vi "RandomLaser.vi"() -> ()   [LabVIEW 2014]
doc: "Random Laser Project\nAndré Romero - 2020\nandretec@ifsc.usp.br\n\nMain Program"
uses:
  OceanOptics.ctl
  PowerMeterSteps.ctl
  RL-Signal.ctl
  <vilib>/Analysis/2dsp.llb/Integral Method.ctl
  <vilib>/Analysis/8numeric.llb/1D Numeric Integration.vi
  GlobalVariables.vi
  <vilib>/Utility/file.llb/Write To Spreadsheet File (DBL).vi
  <vilib>/Analysis/NI_AAL_SigProc.lvlib
  <vilib>/Analysis/NI_AALBase.lvlib
  <vilib>/Analysis/NI_AALPro.lvlib
panel:
  out "delta WL":dbl=0.38690207279938704
  in  "Stop":bool
  out "Power Meter":dbl[](array[numeric])=[-0.0003675591076923077, -0.0002657142871794872, -0.00022899957179487178, 0.00042243897435897433, 0.0004997026012820513, 0.0006796630115384615, 0.000805894673076923, 0.0010408828243589744, 0.0018024533846153848, 0.0023367831153846153, 0.0029247413076923076, 0.0028397148461538463, 0.003205695884615385, 0.0036658875128205127, 0.003961987641025641, 0.004680868307692308, 0.005090419641025641, 0.006488342294871795, 0.007851225423076924, 0.007202216717948717, 0.008655850807692307, 0.008092802884615384, 0.009669394692307692, 0.008936860974358975, 0.009809811717948718, 0.010228137487179488, 0.011672985217948718, 0.012192949025641026, 0.011663994371794871, 0.012874870384615385, 0.01270935917948718, 0.014818592820512821, 0.016178746282051282, 0.016049180384615384, 0.0160890691025641, 0.014186609871794872]
  out "Spectrum":dbl[][](array[numeric])
  out "Amplitudes":dbl[](array[numeric])=[0.0, 0.0, 0.0, 0.0, 0.0, 0.0, 0.0, 0.0, 0.0, 5575.9914689081015, 6701.8830329298, 8561.647140939602, 9059.66238048701, 10013.63040535748, 10875.931356857935, 12579.417450238643, 13233.340345584173, 16127.947959725754, 16741.788066185352, 19933.198034888228, 18892.002085463362, 24420.615194539, 23300.805099557427, 26519.160159321964, 32440.49170739598, 32440.49170739598, 34903.27520346824, 42840.78445676197, 42414.61716171854, 40488.768647175595, 43435.97106846481, 43435.97106846481, 51858.85499836823, 55040.55736237094, 56733.873142532764, 55752.38318456956]
  out "Locations Peaks":dbl[](array[numeric])=[0.0, 0.0, 0.0, 0.0, 0.0, 0.0, 0.0, 0.0, 0.0, 624.9085485139512, 623.199026880973, 622.8569840323327, 622.514895045022, 623.199026880973, 623.199026880973, 622.514895045022, 622.8569840323327, 622.514895045022, 622.8569840323327, 622.514895045022, 622.8569840323327, 622.514895045022, 622.8569840323327, 622.8569840323327, 622.8569840323327, 622.8569840323327, 622.514895045022, 622.514895045022, 622.8569840323327, 622.8569840323327, 622.8569840323327, 622.8569840323327, 622.8569840323327, 622.8569840323327, 622.8569840323327, 622.8569840323327]
  out "Integration":dbl[](array[numeric])=[93876.86248643893, 89574.62293993768, 89574.62293993768, 92418.20959135504, 106316.38021475376, 190489.0806594419, 173427.09120228325, 190883.0319805349, 253633.0446140827, 281236.16658956936, 317841.71014271444, 374352.8298044355, 395197.03367327957, 421997.2274496375, 457040.3478550627, 509121.0411876146, 518774.7267490108, 600545.4510518024, 620849.4391936888, 726021.5293375205, 667303.2962255043, 857398.8951125076, 805420.7981609555, 876101.0180196995, 973816.9103050136, 973816.9103050136, 1101330.125428112, 1300810.123723178, 1183680.9770934903, 1213324.5227469385, 1256065.8933422558, 1256065.8933422558, 1483869.301248752, 1539653.32481904, 1616784.6736414272, 1629926.8709311432]
  out "size(s)":i32=109
  out "Waveform Graph 2":dbl[](graph)=[-0.005487304474358975, -0.005832730371794871, -0.0058483878589743596, -0.0058483878589743596, -0.005573613, -0.005095886692307692, -0.004915247423076923, -0.004803107, -0.004803107, -0.00415237408974359, -0.003636093397435897, -0.003279903192307692, -0.003279903192307692, -0.002614101384615385, -0.002614101384615385, -0.0017563094487179488, -0.0017563094487179488, -0.0006636677525641026, -0.00025933357564102567, -0.00025933357564102567, 0.0005514882038461538, 0.0005514882038461538, 0.001194198632051282, 0.0014312010128205129, 0.0014312010128205129, 0.0027755268974358977, 0.003001960487179487, 0.003001960487179487, 0.003652692653846154, 0.004357635564102564, 0.0060297748717948714, 0.0060297748717948714, 0.006476770166666666, 0.0073061897820512825, 0.008219170974358975, 0.008605500435897437, 0.008900238666666666, 0.010023608461538462, 0.010305812628205128, 0.010305812628205128, 0.012418297, 0.012980169615384615, 0.014193191923076921, 0.013533851282051281, 0.013533851282051281, 0.014171850512820513, 0.01582010935897436, 0.018513849487179487, 0.018513849487179487, 0.020606362692307693, 0.02333670346153846, 0.02333670346153846, 0.022893022307692308, 0.02429118076923077, 0.02429118076923077, 0.02647001435897436, 0.02670231076923077, 0.02670231076923077, 0.027472030897435898, 0.02830790782051282, 0.02830790782051282, 0.02888465923076923, 0.03174886423076923, 0.03174886423076923, 0.032283935897435896, 0.03257239217948718, 0.03271840076923077, 0.03444572064102564, 0.034723633846153845, 0.034723633846153845, 0.03663491371794872, 0.03663491371794872, 0.03613761141025641, 0.03828260551282051, 0.03805538666666667, 0.03805538666666667, 0.03951163782051282, 0.04004338717948718, 0.039338835769230765, 0.039338835769230765, 0.04283988615384615, 0.042323017051282046, 0.042323017051282046, 0.04017059935897436, 0.04026514051282051, 0.041000410641025636, 0.041000410641025636, 0.04617789256410257, 0.04617789256410257, 0.046548361923076924, 0.04826218653846154, 0.04826218653846154, 0.048524028461538464, 0.04702962294871795, 0.04661353666666666, 0.04663584961538462, 0.04663584961538462, 0.0458491058974359, 0.04640453230769231, 0.04640453230769231, 0.04648593948717949, 0.04691024641025641, 0.04691024641025641, 0.04794475782051282, 0.04896243064102564, 0.05036391884615385, 0.05036391884615385, 0.04973549115384615, 0.04851584358974359]
  out "Motor Target":i32
  out "step error":dbl=4.6948184809657505
  out "Numeric Control":i32=571
  out "appended array":dbl[](array[numeric])=[0.03814716076923077, 0.04028040576923077, 0.03893296115384615, 0.03881278179487179, 0.03962595474358974, 0.03962595474358974, 0.04072623166666667, 0.042531442307692305, 0.042531442307692305, 0.04118947217948718, 0.04118947217948718, 0.043604905, 0.04170907846153846, 0.047686999358974365, 0.04542324666666667, 0.04744549717948718, 0.04744549717948718, 0.04903151871794872, 0.04903151871794872, 0.05148572076923077, 0.05148572076923077, 0.04996409794871795, 0.04996409794871795, 0.05131271576923077, 0.052321403717948724, 0.05075768333333334, 0.0506429873076923, 0.05160921064102564, 0.04980653423076923, 0.04980653423076923, 0.05041557743589743, 0.050435350128205124, 0.05207693756410257, 0.0510150267948718, 0.04899962987179487, 0.05028836243589744, 0.05107413, 0.05107413, 0.047357233589743586, 0.05035041474358974, 0.050845735, 0.050845735, 0.049560324871794875, 0.049386343589743587, 0.049386343589743587, 0.0474762308974359, 0.05124815, 0.05124815, 0.04991651987179487, 0.047606959358974354, 0.046334271153846154, 0.047763528974358975, 0.047946701025641025, 0.04803633192307692, 0.04881388474358974, 0.04784396294871795, 0.04784396294871795, 0.04528820487179487, 0.04316417756410257, 0.04157324871794872, 0.04189031333333333, 0.04189031333333333, 0.042249424743589746, 0.042249424743589746, 0.04073130923076923, 0.038956053205128204, 0.038956053205128204, 0.04025163923076923, 0.040992975, 0.03823464833333333, 0.037050615, 0.03659950551282051, 0.035411361794871796, 0.035411361794871796, 0.0335793308974359, 0.032886507564102566, 0.032659309615384616, 0.031678015000000004, 0.031678015000000004, 0.030108811153846154, 0.030108811153846154, 0.02815076512820513, 0.027613132307692308, 0.02745461641025641, 0.02745461641025641, 0.024971846153846153, 0.023404218333333334, 0.023404218333333334, 0.022565616153846155, 0.021971435384615386, 0.021303487435897436, 0.020184618333333335, 0.019698665, 0.019698665, 0.01710024217948718, 0.016112891025641025, 0.016112891025641025, 0.01559681141025641, 0.01566960833333333, 0.014254835256410258, 0.01331249358974359, 0.01331249358974359, 0.01175093273076923, 0.011184945320512821, 0.010219515294871796, 0.009239205, 0.008537592243589744, 0.008537592243589744, 0.008233652730769231, 0.007168407769230769, 0.007049413397435898, 0.006302984474358974, 0.0051921379102564105, 0.00454199676923077, 0.003954869897435898, 0.003954869897435898, 0.0031781009743589743, 0.0031781009743589743, 0.0029140872564102564, 0.0014977446794871795, 0.0014977446794871795, 0.0006180309871794871, -0.0002421096346153846, -0.0002421096346153846, -0.0010443222076923077, -0.0010443222076923077, -0.0019091590384615385, -0.0027440524102564103, -0.0027949365512820513, -0.0028524740769230767, -0.003429424858974359, -0.0048430307435897435, -0.004761224730769231, -0.004563362333333334, -0.004991378192307692, -0.004588804679487179, -0.004029664871794872, -0.003666037141025641, -0.003666037141025641, -0.003410441705128205, -0.002968921858974359, -0.002852083217948718, -0.002779084102564103, -0.002779084102564103, -0.002142247705128205, -0.0018751047564102563, -0.0018751047564102563, -0.0015238072564102564, -0.0011774021769230768, -0.0008895146423076923, -0.0006176758641025641, -0.00047911462564102563, -0.00047911462564102563, -0.0003826308576923077, -0.0013799610128205127, -0.0005440882743589744, -0.00013818675897435897, -0.00013818675897435897, 0.0018592164999999999, 0.0027060513974358972, 0.0034595305384615385, 0.0034595305384615385, 0.004154488961538461, 0.005114832538461538, 0.005114832538461538, 0.0064566116538461536, 0.006633336833333333, 0.006633336833333333, 0.006688135615384616, 0.007803289166666667, 0.007803289166666667, 0.009279321282051282, 0.009510256435897436, 0.009510256435897436, 0.010018718269230769, 0.011323302692307692, 0.013602139358974358, 0.013602139358974358, 0.014472458846153847, 0.014472458846153847, 0.015263318846153848, 0.016187063974358974, 0.01790519141025641, 0.01790519141025641, 0.019298054487179486, 0.019298054487179486, 0.020291468205128206, 0.020291468205128206, 0.021376090384615385, 0.021376090384615385, 0.02242841923076923, 0.023227692435897434, 0.025591651794871793, 0.025591651794871793, 0.026223805, 0.02971779294871795, 0.028628870897435897, 0.028628870897435897, 0.028008663717948717, 0.027696697564102566, 0.02956965, 0.02956965, 0.028673496794871793, 0.029780030384615387, 0.03213930923076923, 0.035217996025641025, 0.03527473807692308, 0.03527473807692308, 0.03669559897435897, 0.03665665358974359, 0.03785556128205128, 0.03754203987179487, 0.036888361794871795, 0.037945386153846156, 0.03861492346153846, 0.038500227435897434, 0.03922416064102564, 0.040526400384615385, 0.040526400384615385, 0.03986666282051282, 0.03986666282051282, 0.04169341923076923, 0.041507686025641026, 0.042650239743589745, 0.04226409, 0.04226409, 0.04266863628205128, 0.0441421408974359, 0.04573343076923077, 0.04521813487179487, 0.047250176153846156, 0.047250176153846156, 0.04542147653846154, 0.04631489551282051, 0.048990803205128206, 0.047789943333333335, 0.047789943333333335, 0.04684231358974359, 0.04454275576923077, 0.04685368358974359, 0.04762596192307692, 0.04675973038461539, 0.04675973038461539, 0.04527703205128205, 0.04527703205128205, 0.04157364871794872, 0.041092978846153844, 0.041092978846153844, 0.041301809999999994, 0.042665305, 0.04386481269230769, 0.04386481269230769, 0.04428675551282051, 0.0458058591025641, 0.046089819871794876, 0.046089819871794876, 0.046192972820512816, 0.0462835708974359, 0.044576599871794874, 0.044576599871794874, 0.04427247525641026, 0.04392391884615385, 0.04286120217948718, 0.04286120217948718, 0.04098240512820513, 0.04072601384615385, 0.03965080487179487, 0.03965080487179487, 0.0398696, 0.039303415641025644, 0.04005141987179487, 0.04017236935897436, 0.0395265241025641, 0.03754184576923077, 0.03754184576923077, 0.03593919487179487, 0.03592997423076923, 0.03364331756410256, 0.03334448538461539, 0.033942364615384614, 0.031980772435897434, 0.03136175038461538, 0.02979686871794872, 0.02979686871794872, 0.027415076923076924, 0.02804057653846154, 0.026967289871794874, 0.026967289871794874, 0.023854156153846156, 0.023854156153846156, 0.02363947141025641, 0.023173087692307692, 0.02205128576923077, 0.02286054987179487, 0.022448578461538464, 0.022448578461538464, 0.02149762794871795, 0.02094963717948718, 0.019584764487179485, 0.018592137307692307, 0.017544697948717946, 0.01551637141025641, 0.014312563846153847, 0.014088873333333331, 0.013259848461538461, 0.012367222012820513, 0.012367222012820513, 0.011250896833333333, 0.01044046858974359, 0.009141736282051283, 0.009141736282051283, 0.007557283448717949, 0.007557283448717949, 0.007006557628205129, 0.006270297884615385, 0.006270297884615385, 0.004901510038461538, 0.004901510038461538, 0.004756689756410257, 0.004255871782051282, 0.0034951461666666663, 0.0031088181794871796, 0.0025083835897435898, 0.0021981839615384615, 0.001356832141025641, 0.001356832141025641, 0.0003710442217948718, -0.00028144756666666665, -0.0007325553064102564, -0.0011335642525641025, -0.0011335642525641025, -0.001437696576923077, -0.0018406603717948718, -0.0018406603717948718, -0.002247147051282051, -0.002247147051282051, -0.0023632034230769232, -0.002725851705128205, -0.002725851705128205, -0.00294974317948718, -0.003120204871794872, -0.003120204871794872, -0.0034253148846153845, -0.0036460745256410255, -0.0055601084487179485, -0.005810028641025641, -0.00561432067948718, -0.005487304474358975, -0.005487304474358975, -0.005832730371794871, -0.0058483878589743596, -0.0058483878589743596, -0.005573613, -0.005095886692307692, -0.004915247423076923, -0.004803107, -0.004803107, -0.00415237408974359, -0.003636093397435897, -0.003279903192307692, -0.003279903192307692, -0.002614101384615385, -0.002614101384615385, -0.0017563094487179488, -0.0017563094487179488, -0.0006636677525641026, -0.00025933357564102567, -0.00025933357564102567, 0.0005514882038461538, 0.0005514882038461538, 0.001194198632051282, 0.0014312010128205129, 0.0014312010128205129, 0.0027755268974358977, 0.003001960487179487, 0.003001960487179487, 0.003652692653846154, 0.004357635564102564, 0.0060297748717948714, 0.0060297748717948714, 0.006476770166666666, 0.0073061897820512825, 0.008219170974358975, 0.008605500435897437, 0.008900238666666666, 0.010023608461538462, 0.010305812628205128, 0.010305812628205128, 0.012418297, 0.012980169615384615, 0.014193191923076921, 0.013533851282051281, 0.013533851282051281, 0.014171850512820513, 0.01582010935897436, 0.018513849487179487, 0.018513849487179487, 0.020606362692307693, 0.02333670346153846, 0.02333670346153846, 0.022893022307692308, 0.02429118076923077, 0.02429118076923077, 0.02647001435897436, 0.02670231076923077, 0.02670231076923077, 0.027472030897435898, 0.02830790782051282, 0.02830790782051282, 0.02888465923076923, 0.03174886423076923, 0.03174886423076923, 0.032283935897435896, 0.03257239217948718, 0.03271840076923077, 0.03444572064102564, 0.034723633846153845, 0.034723633846153845, 0.03663491371794872, 0.03663491371794872, 0.03613761141025641, 0.03828260551282051, 0.03805538666666667, 0.03805538666666667, 0.03951163782051282, 0.04004338717948718, 0.039338835769230765, 0.039338835769230765, 0.04283988615384615, 0.042323017051282046, 0.042323017051282046, 0.04017059935897436, 0.04026514051282051, 0.041000410641025636, 0.041000410641025636, 0.04617789256410257, 0.04617789256410257, 0.046548361923076924, 0.04826218653846154, 0.04826218653846154, 0.048524028461538464, 0.04702962294871795, 0.04661353666666666, 0.04663584961538462, 0.04663584961538462, 0.0458491058974359, 0.04640453230769231, 0.04640453230769231, 0.04648593948717949, 0.04691024641025641, 0.04691024641025641, 0.04794475782051282, 0.04896243064102564, 0.05036391884615385, 0.05036391884615385, 0.04973549115384615, 0.04851584358974359, 0.04851584358974359, 0.04918926448717949, 0.04918926448717949, 0.04768798435897436, 0.04749853782051282, 0.045149443846153846, 0.04514924974358975, 0.04693097435897436, 0.04693097435897436, 0.04631743282051282, 0.044912025256410255, 0.04394035730769231, 0.04564164179487179, 0.04489031230769231, 0.04489031230769231, 0.04320840641025641, 0.041405327051282054, 0.03952789717948718, 0.03952789717948718, 0.04017042025641026, 0.03891552269230769, 0.03727723974358974, 0.03727723974358974, 0.03708113961538462, 0.035381607307692305, 0.03470992666666667, 0.03470992666666667, 0.033015304615384614, 0.0317245991025641, 0.03036636948717949, 0.03337051474358974, 0.031271919615384614, 0.031271919615384614, 0.03185395435897436, 0.029991192820512817, 0.029809205769230768, 0.030315111025641026, 0.030740970128205126, 0.02854235935897436, 0.02854235935897436, 0.028143314487179487, 0.02606488012820513, 0.025311992435897435, 0.025311992435897435, 0.025301225512820512, 0.026598984615384614, 0.023089526923076923, 0.02366060076923077, 0.021547534358974357, 0.020616556538461537, 0.01807409358974359, 0.01857530782051282, 0.01828310987179487, 0.01758873730769231, 0.01758873730769231, 0.016613126153846153, 0.01586845166666667, 0.014894025512820513, 0.014096111923076924, 0.013694126794871794, 0.013694126794871794, 0.012646690423076925, 0.01233981964102564, 0.011144820089743589, 0.011144820089743589, 0.007031992141025642, 0.007031992141025642, 0.006841767269230769, 0.006366588282051282, 0.005964797217948718, 0.005393916628205128, 0.005393916628205128, 0.0047112851666666665, 0.0047112851666666665, 0.004555888243589743, 0.004352743512820513, 0.003906722833333333, 0.0028285643461538465, 0.0028285643461538465, 0.0023823483333333334, 0.0014584036666666666, 0.0014584036666666666, 0.0009810724012820514, 6.065033628205128e-05, -0.0003385933807692308, -0.0007675893217948718, -0.0012159566371794871, -0.0012159566371794871, -0.0019612159102564103, -0.0020081876282051284, -0.0023172115384615384, -0.002345588884615385, -0.0023684878205128203, -0.002424069230769231, -0.002487282564102564, -0.002487282564102564, -0.0024958937564102564, -0.0024958937564102564, -0.002623887730769231, -0.002822531076923077, -0.0029495465384615383, -0.002981251807692308, -0.0028888769999999998, -0.0029963206923076923, -0.0029963206923076923, -0.0031554324487179488, -0.0030192192435897435, -0.0028800697307692306, -0.0031667833205128205, -0.003918306153846154, -0.004110883217948718, -0.004110883217948718, -0.0034198355256410255, -0.0031898775769230773, -0.001915811128205128]
  out "Locations":dbl[](array[numeric])=[133.6766422737507, 347.8606807155645, 566.3051815190342]
  out "Amplitudes":dbl[](array[numeric])=[-0.004824217477593765, -0.0057485308347034105, -0.0038350874887697647]
  out "standard deviation":dbl=3.0126018269169577 format="%0.2f"
  out "mean":dbl=216.31426962264177 format="%0.2f"
  out "Array":dbl[](array[numeric])=[214.1840384418138, 218.44450080346974]
  out "# found":i32=3
  in  "Select Light Source":u16(ring)=6
  in  "Tab Control":T1(tab)=enum."Settings"
  in  "Range List":T2(array[cluster])=[{"Name"="Sample", "Inicial"=500.0, "Final"=700.0}]
  out "Current Position":dbl=36.0
  out "Min power to Aqc":dbl
  out "Max power to Aqc":dbl
  out "Low power":bool
  out "Max power":bool
  in  "Clear Dark Spec":bool caption="Blank Button"
  in  "Average":i32=2
  in  "Integration Time":i32=100
  out "Spectrum":T3(graph)
  in  "Store Dark Spec":bool caption="Blank Button"
  in  "threshold":dbl=5000.0 format="%0.2f"
  in  "width":i32=10 min=3
  out "Power Meter [W]":dbl format="%#_4p"
  in  "Power up":bool
  in  "Power down":bool
  in  "Half Power":bool
  in  "min Power":bool
  in  "max Power Go":bool
  out "Max Power":dbl=0.052321403717948724 format="%#_3p"
  out "Min Power":dbl=-0.0058483878589743596 format="%#_3p"
  in  "Correct Electrical Dark":bool
  out "table":string[][](table)=[["Name", "Integration", "Peak", "WL"], ["Sample", "1734", "0", "0,00"]]
  out "Power Meter":dbl format="%#_4p"
  in  "Tuning Motor":bool
  out "Power Meter":dbl(graph)=-0.001915811128205128
  out "Min Power":dbl=-0.0058483878589743596 format="%#_3p"
  out "Max Power":dbl=0.052321403717948724 format="%#_3p"
  out "Power Meter [W]":dbl format="%#_4p"
  out "Running":bool
  in  "Step Stop":i32=35
  in  "Save Aquisition":bool
  in  "Play Aquisition":bool
  out "Sample":cluster{dbl[], dbl[]}(graph)={[-0.0003675591076923077, -0.0002657142871794872, -0.00022899957179487178, 0.00042243897435897433, 0.0004997026012820513, 0.0006796630115384615, 0.000805894673076923, 0.0010408828243589744, 0.0018024533846153848, 0.0023367831153846153, 0.0029247413076923076, 0.0028397148461538463, 0.003205695884615385, 0.0036658875128205127, 0.003961987641025641, 0.004680868307692308, 0.005090419641025641, 0.006488342294871795, 0.007851225423076924, 0.007202216717948717, 0.008655850807692307, 0.008092802884615384, 0.009669394692307692, 0.008936860974358975, 0.009809811717948718, 0.010228137487179488, 0.011672985217948718, 0.012192949025641026, 0.011663994371794871, 0.012874870384615385, 0.01270935917948718, 0.014818592820512821, 0.016178746282051282, 0.016049180384615384, 0.0160890691025641, 0.014186609871794872], [0.0, 0.0, 0.0, 0.0, 0.0, 0.0, 0.0, 0.0, 0.0, 5575.9914689081015, 6701.8830329298, 8561.647140939602, 9059.66238048701, 10013.63040535748, 10875.931356857935, 12579.417450238643, 13233.340345584173, 16127.947959725754, 16741.788066185352, 19933.198034888228, 18892.002085463362, 24420.615194539, 23300.805099557427, 26519.160159321964, 32440.49170739598, 32440.49170739598, 34903.27520346824, 42840.78445676197, 42414.61716171854, 40488.768647175595, 43435.97106846481, 43435.97106846481, 51858.85499836823, 55040.55736237094, 56733.873142532764, 55752.38318456956]}
  in  "correction factor":dbl=0.078
  out "Power Value":dbl caption="Optical Power [W]" format="%#_4p"
  in  "Average Time (0.0)":dbl=0.5
  out "P Meter Delay (ms)":u32=1
  out "Spectrum delay (ms)":u32=206
  # "Set power to Aquisition"
  # "Move Step Motor"
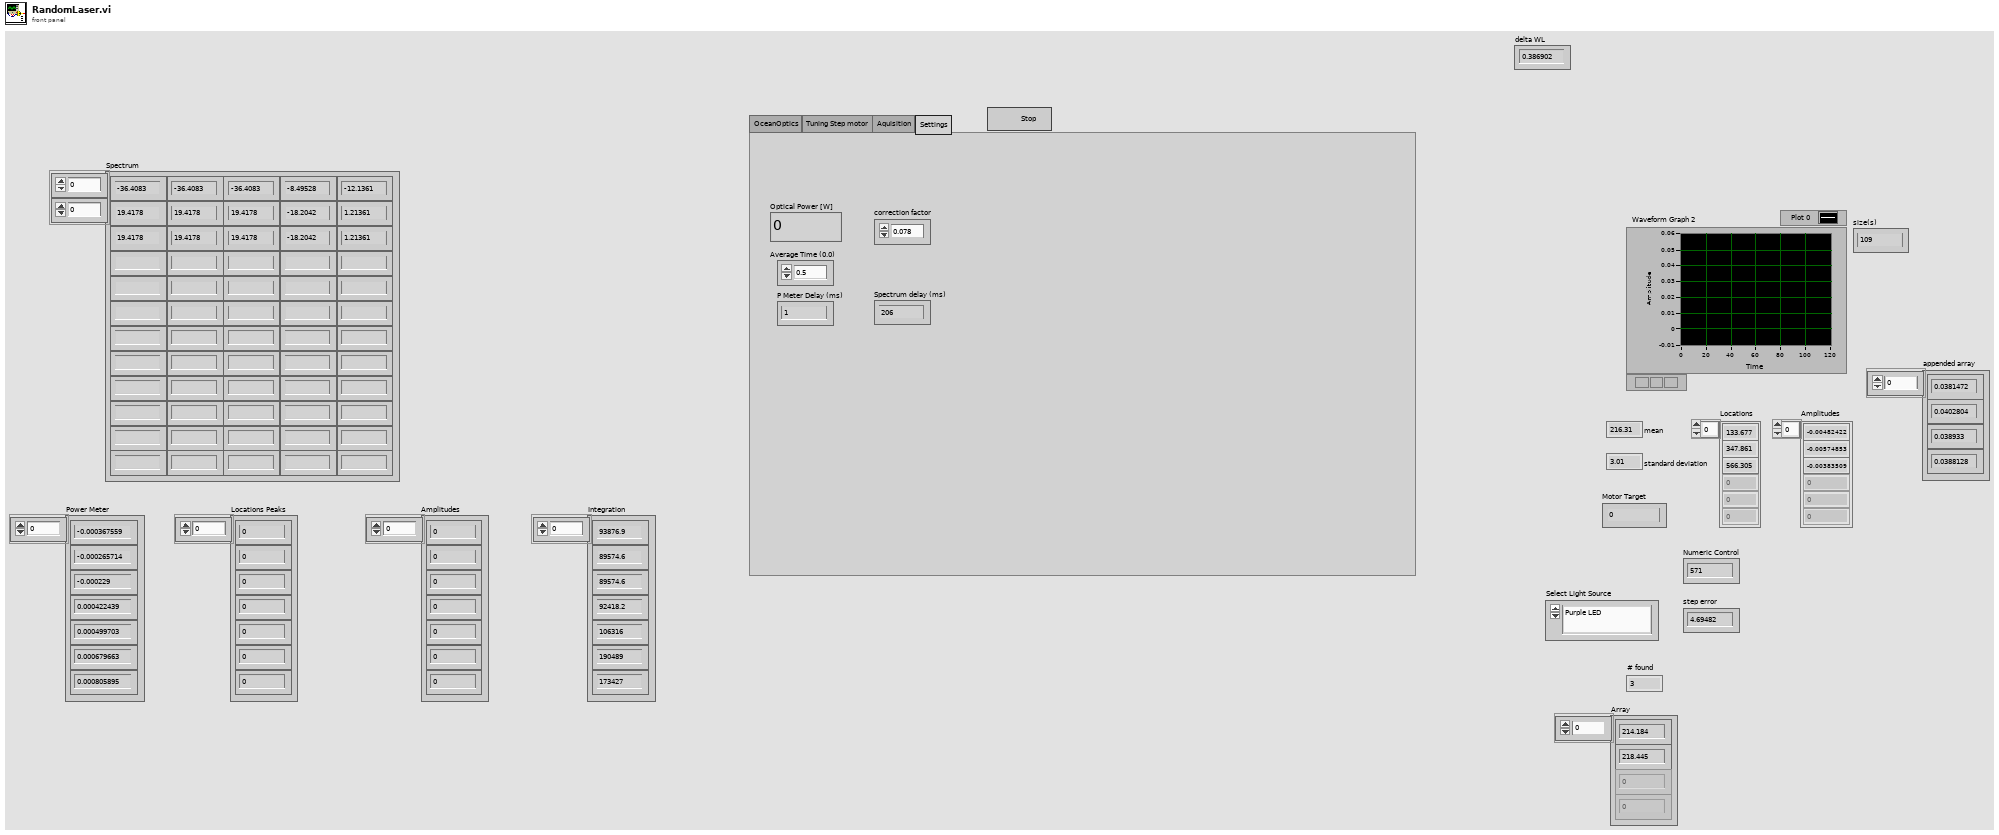
[diagram p1: front panel]
types:
  T1 = enum32{"OceanOptics", "Tuning Step motor", "Aquisition", "Settings"}
  T2 = cluster{"Name":string, "Inicial":dbl, "Final":dbl}[]
  T3 = cluster{"WL Values":dbl[], "Spectrum Values":dbl[]}[]
  T4 = typedef "PowerMeterSteps.ctl" = enum16{"Initialize", "Graph", "Wait for Event", "Tuning", "Get Power", "MoveMotor", "corrects step"}
  T5 = typedef "OceanOptics.ctl" = enum16{"Initialize", "Graph", "Wait for Event", "Dark Spec", "Clear Dark Spec", "OceanOptics", "Create File", "Save"}
  T6 = enum16{"open", "replace", "create", "open or create", "replace or create", "replace or create with confirmation"}
  T7 = typedef "RL-Signal.ctl" = cluster{"Signal State":string, "Step":dbl, "Integration value":dbl, "Peak value":dbl, "Peak Wavelenght":dbl, "Spectrum values ":dbl[], "Error":errorcluster}
  T8 = cluster{"WL Values":dbl[], "Spectrum Values":dbl[]}
  T9 = cluster{"Wavelenght":dbl[], "Spectrum Values":dbl[]}
  T10 = typedef "NI_AALPro.lvlib/Integral Method.ctl" = i32
  T11 = cluster{"Wavelenght":dbl[], "Spectrum Values":dbl[]}[]
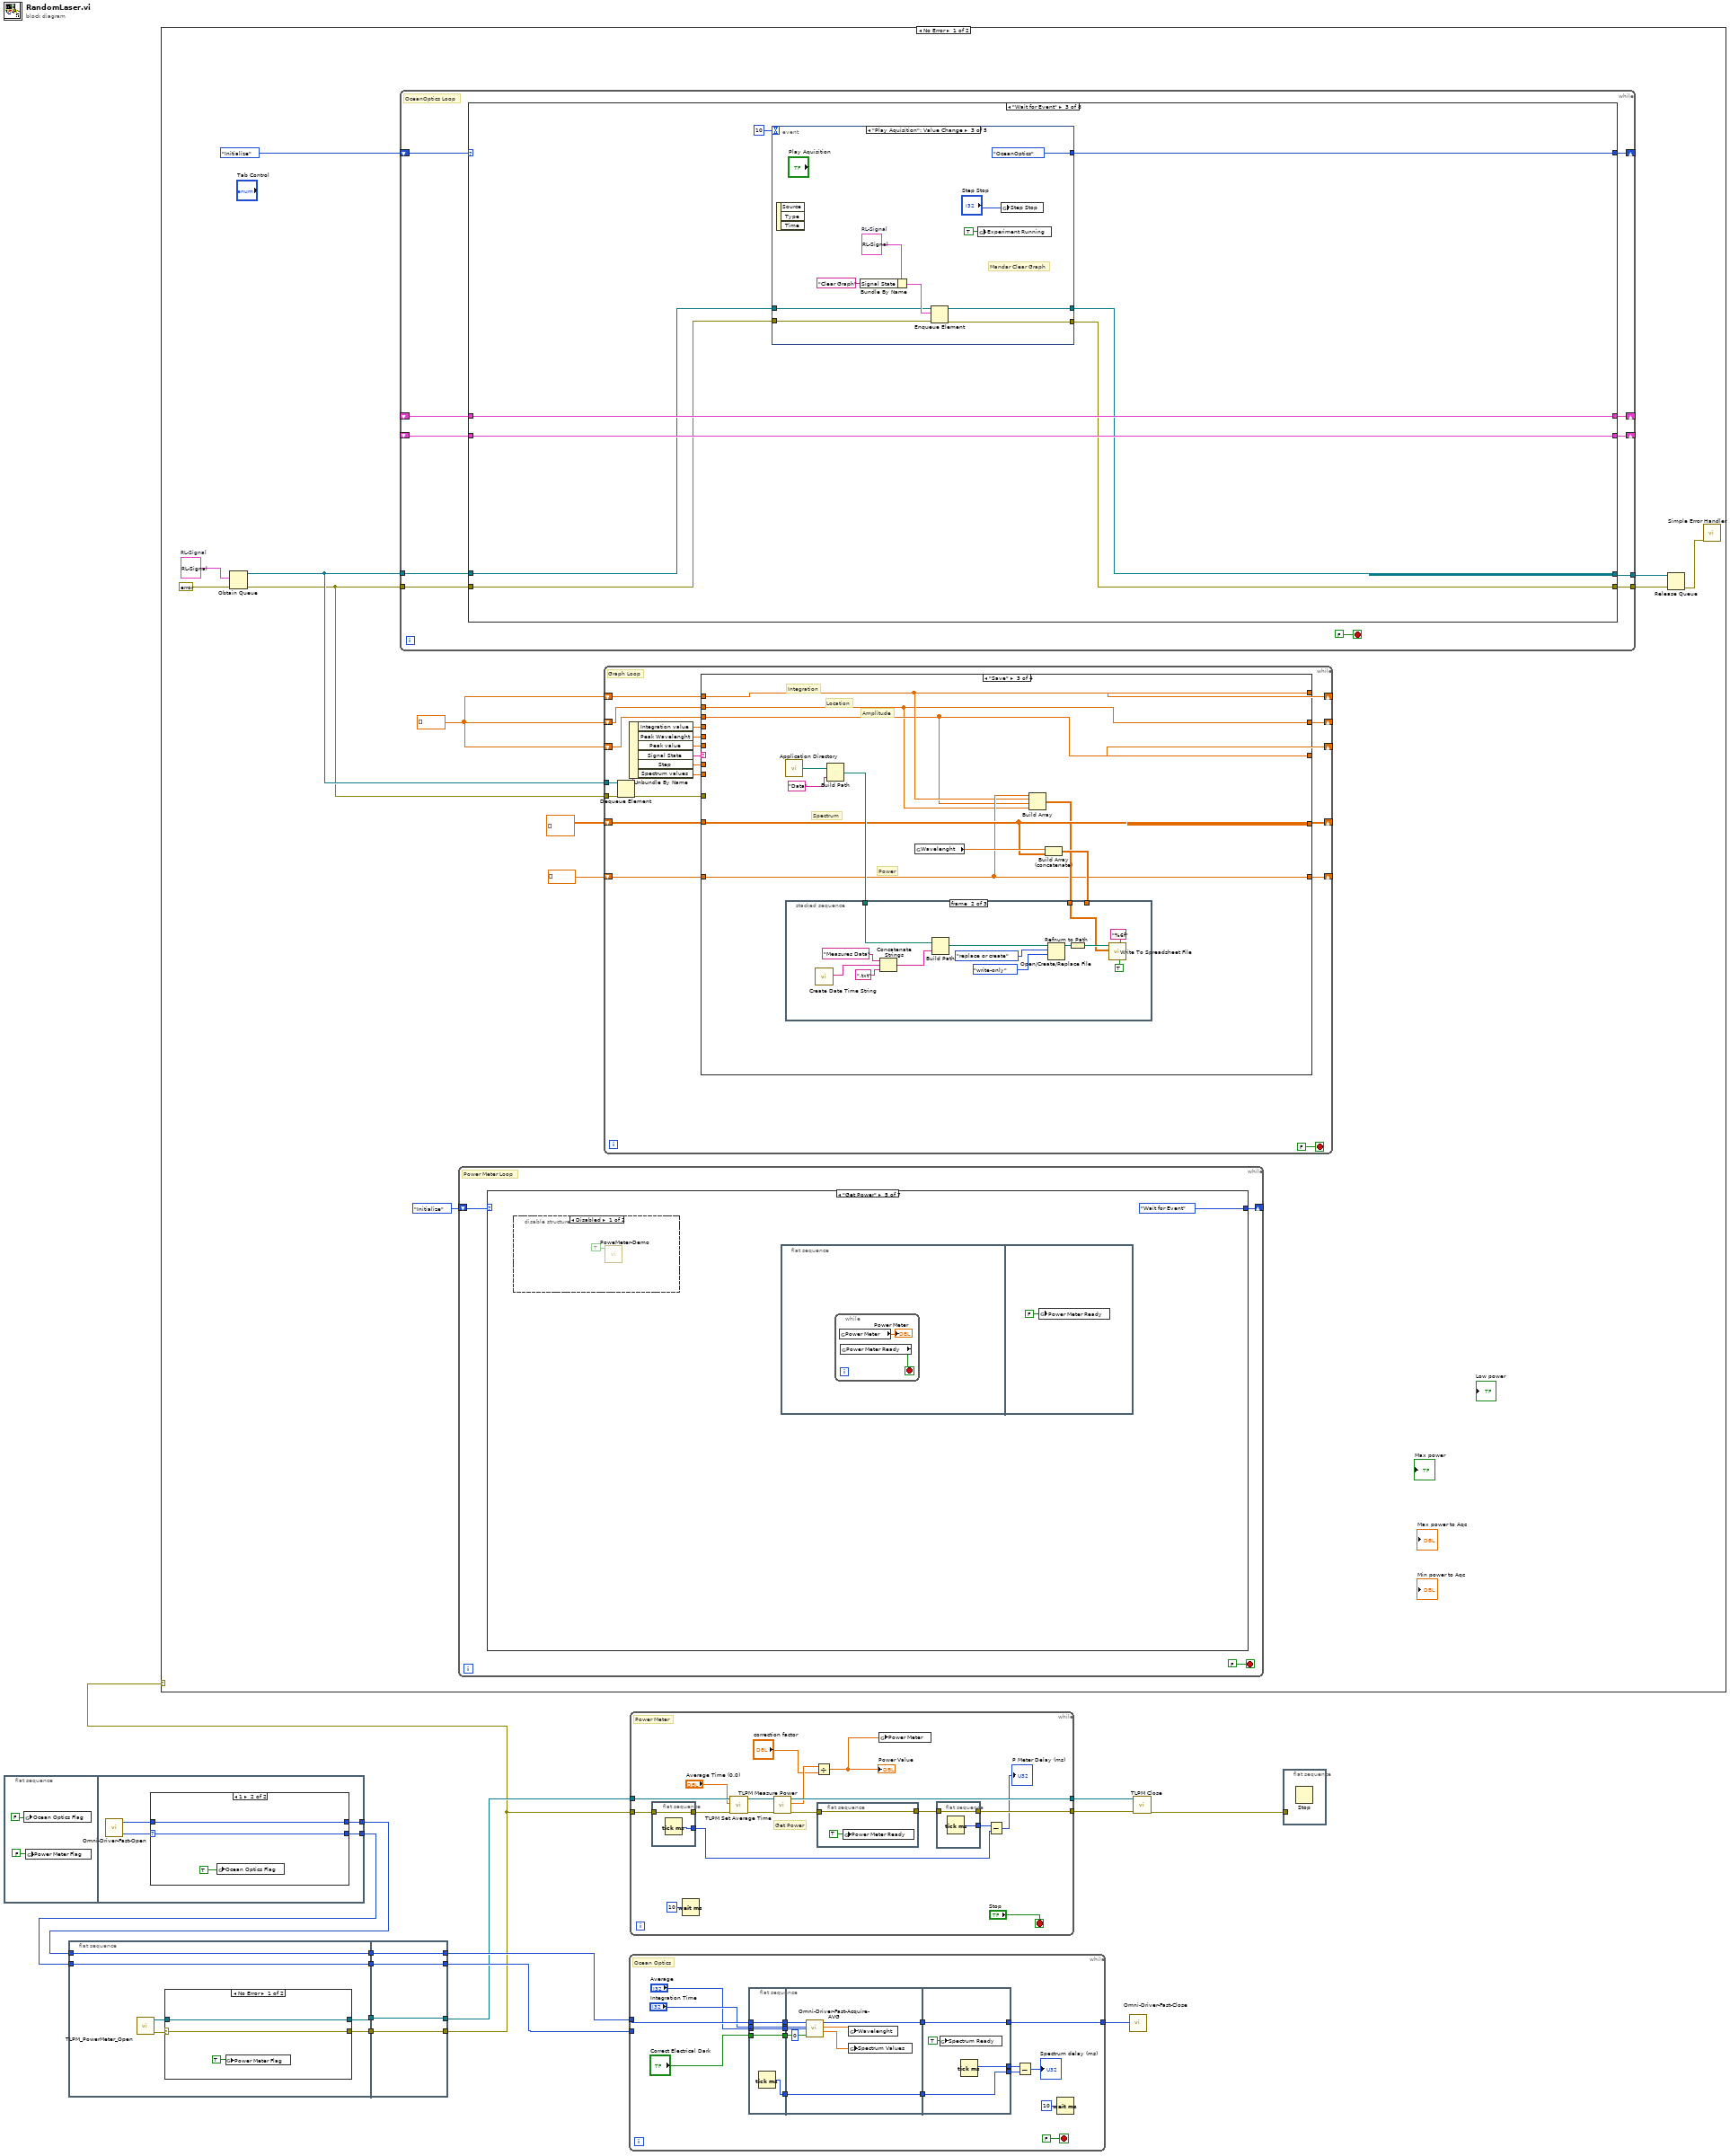
[diagram p0: block diagram]
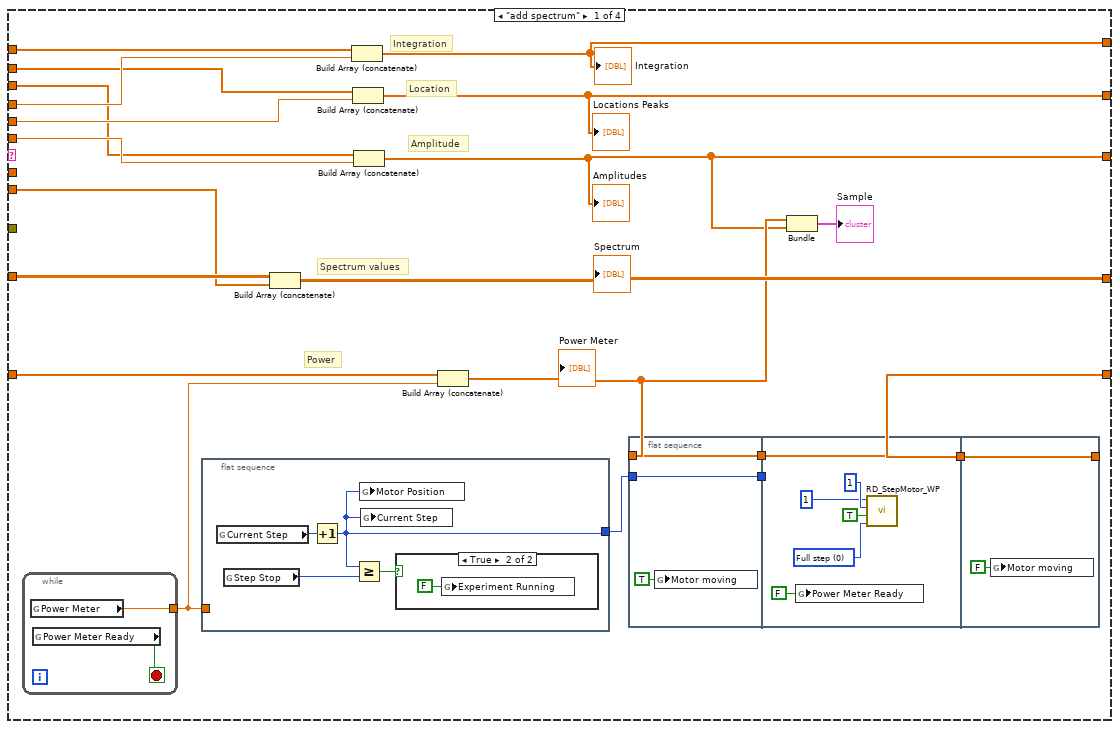
[diagram p2: hidden frame]
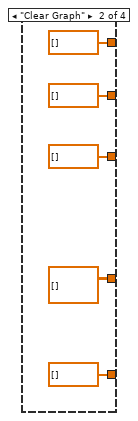
[diagram p4: hidden frame]
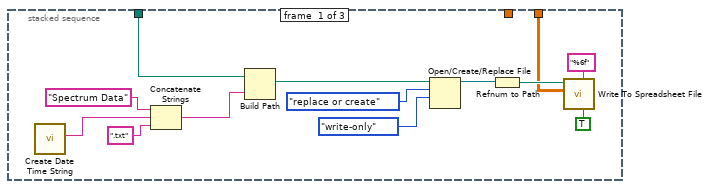
[diagram p5: hidden frame]
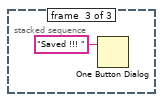
[diagram p6: hidden frame]
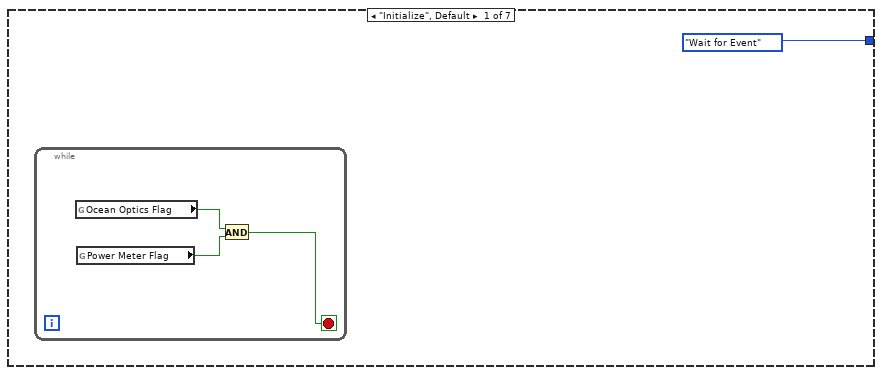
[diagram p8: hidden frame]
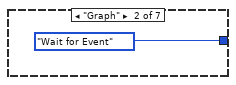
[diagram p9: hidden frame]
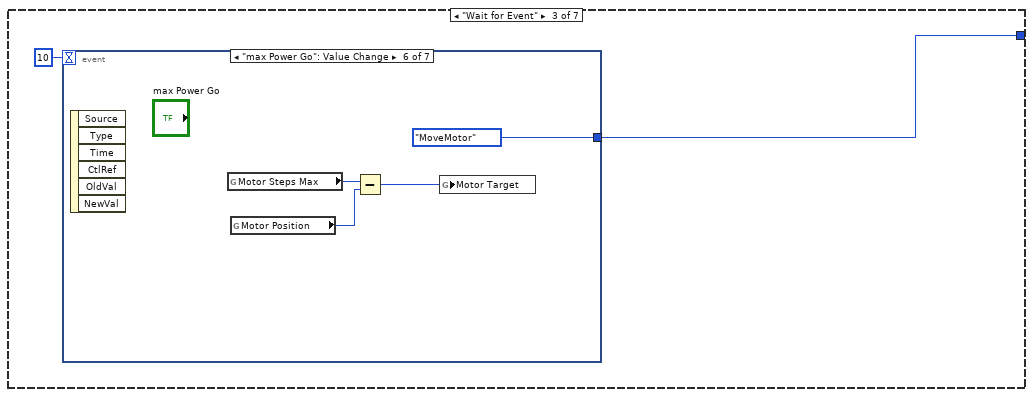
[diagram p10: hidden frame]
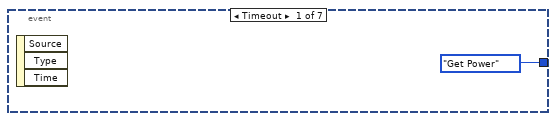
[diagram p11: hidden frame]
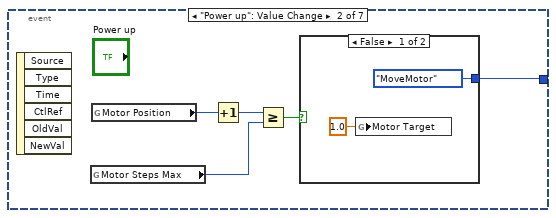
[diagram p12: hidden frame]
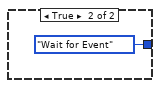
[diagram p13: hidden frame]
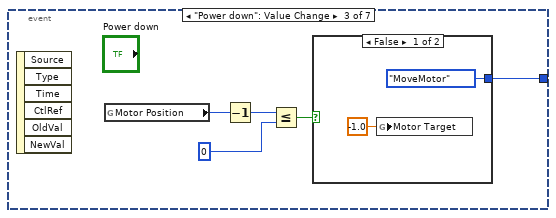
[diagram p14: hidden frame]
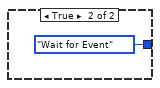
[diagram p15: hidden frame]
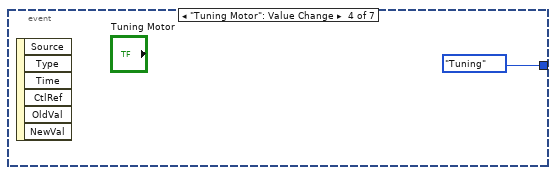
[diagram p16: hidden frame]
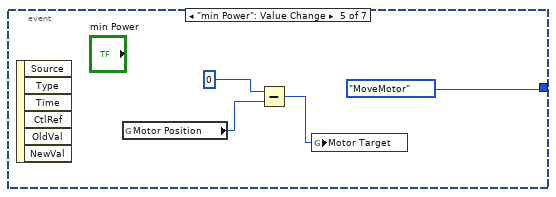
[diagram p17: hidden frame]
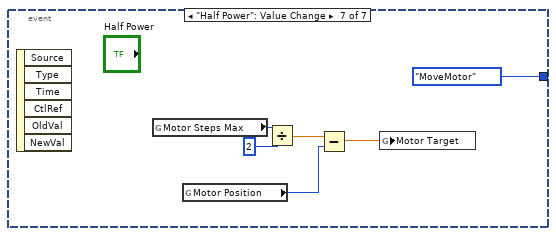
[diagram p18: hidden frame]
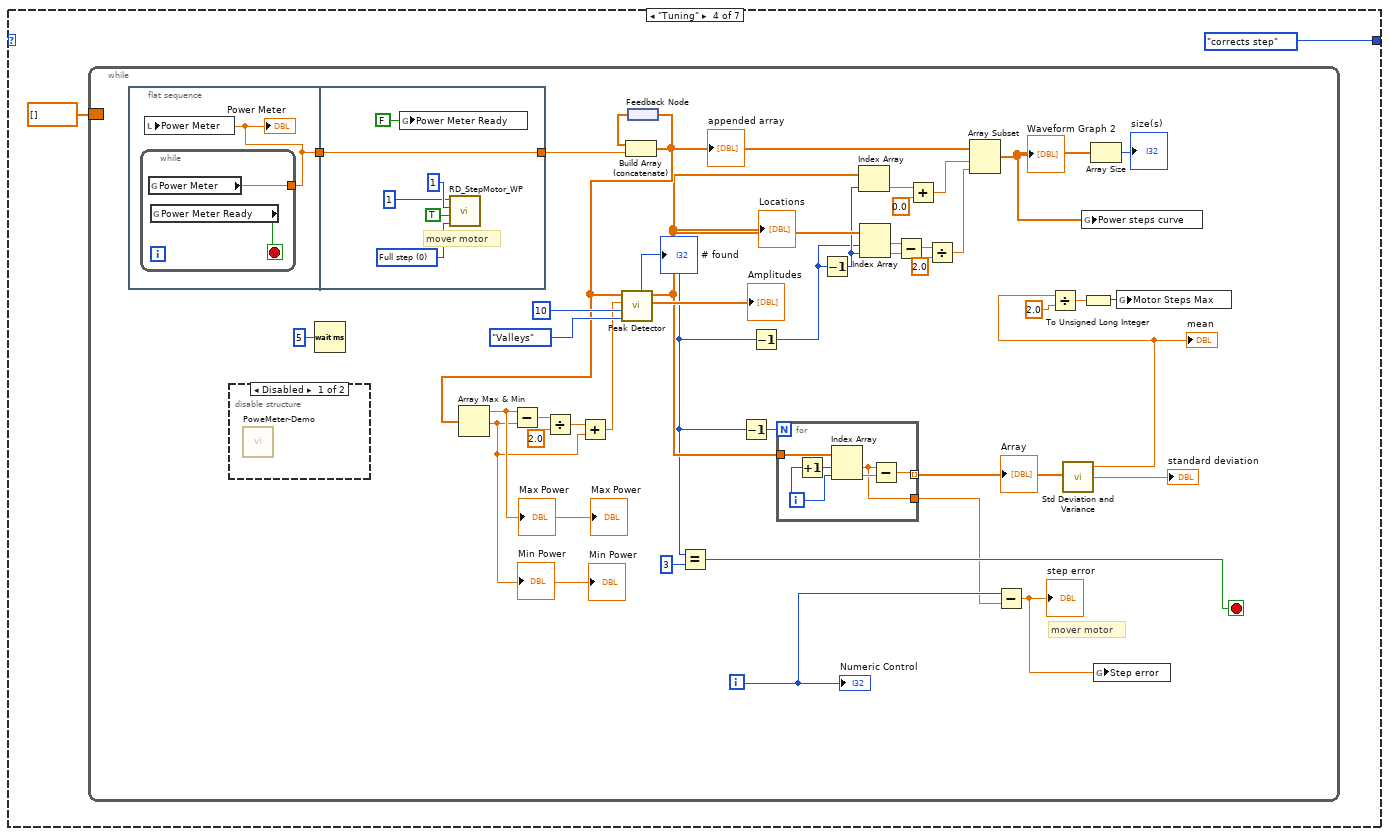
[diagram p19: hidden frame]
diagram:
  n1 = flat-sequence {
    tunnel: [w18] -> w8
    tunnel: [w17] -> w7
    frame #0 {
      n2 = global write "GlobalVariables.vi" "Ocean Optics Flag"(FALSE ("Ocean Optics")) -> ()
      n3 = global write "GlobalVariables.vi" "Power Meter Flag"(FALSE ("Ocean Optics")) -> ()
    }
    frame #1 {
      n4 = call "Omni-Driver-Fast-Open.vi"() -> ("Number of Spectrometers"=w20:i32, "Wrapper Out"=w19:u32)  [unwired: 4 in]
      n5 = case shown="1" w20 {
        selector: w20 -> [_ w23]
        tunnel: w19 -> [_ w24]
        tunnel: [_ w24] -> w18
        tunnel: [_ w23] -> w17
        frame 0, Default {
          n6 = flat-sequence {
            frame #0 {
              n7 = One Button Dialog(message="Ocean Optics not Connected") -> ()  [unwired: 1 in, 1 out]
            }
            frame #1 {
              n8 = Stop() -> ()  [unwired: 1 in]
            }
          }
        }
        frame 1 {
          n9 = global write "GlobalVariables.vi" "Ocean Optics Flag"(TRUE ("Ocean Optics")) -> ()
        }
      }
    }
  }
  n10 = flat-sequence {
    tunnel: [w28] -> w10
    tunnel: [w27] -> w9
    tunnel: w8 -> [w26]
    tunnel: w7 -> [w25]
    tunnel: [w26] -> w6
    tunnel: [w25] -> w3
    tunnel: w10 -> [w38]
    tunnel: [w38] -> w2
    tunnel: [w37] -> w1
    tunnel: w9 -> [w37]
    tunnel: [w36] -> w5
    tunnel: w6 -> [w36]
    tunnel: [w35] -> w4
    tunnel: w3 -> [w35]
    frame #0 {
      n11 = call "TLPM_PowerMeter_Open.vi"() -> ("error out"=w30:errorcluster, "instrument handle out"=w29:refnum<visa-resource-name>)  [unwired: 10 in]
      n12 = case shown="No Error" w30 {
        selector: w30 -> [w32 _]
        tunnel: w29 -> [w33 _]
        tunnel: [w33 _] -> w28
        tunnel: [w32 _] -> w27
        frame No Error {
          n13 = global write "GlobalVariables.vi" "Power Meter Flag"(TRUE ("Ocean Optics")) -> ()
        }
        frame Error {
          n14 = flat-sequence {
            frame #0 {
              n15 = One Button Dialog(message="Power Meter not Connected") -> ()  [unwired: 1 in, 1 out]
            }
            frame #1 {
              n16 = Stop() -> ()  [unwired: 1 in]
            }
          }
        }
      }
    }
    frame #1 {
    }
  }
  n17 = case shown="No Error" w1 {
    frame No Error {
      w43 = dbl[] []
      w47 = T7 {"Signal State"="", "Step"=0.0, "Integration value"=0.0, "Peak value"=0.0, "Peak Wavelenght"=0.0, "Spectrum values "=[], "Error"={"status"=FALSE, "code"=0, "source"=""}}  # RL-Signal
      n18 = Obtain Queue(element data type=w47, error in (no error)=errorcluster {"status"=FALSE, "code"=0, "source"=""}) -> (queue out=w46:refnum<queue>, error out=w45:errorcluster)  [unwired: 3 in, 1 out]
      n19 = while {
        shift-right: [w292] -> _
        shift-left: OceanOptics."Initialize" -> [w289]
        shift-right: [w295] -> _
        shift-left: _ -> [w294]
        shift-right: [w291] -> _
        shift-left: _ -> [w290]
        tunnel: w45 -> [w288]
        tunnel: w46 -> [w287]
        tunnel: [w286] -> w40
        tunnel: [w285] -> w39
        stop <- FALSE stop-if-true
        # "OceanOptics Loop"
        n20 = case shown="\"Wait for Event\"" w289 {
          tunnel: [w299 w308 w316 w376 w448 w453 w456 w466] -> w295
          tunnel: w294 -> [_ w308 w316 _ w448 w453 w456 w466]
          tunnel: [OceanOptics."OceanOptics" OceanOptics."OceanOptics" w315 w379 OceanOptics."OceanOptics" OceanOptics."OceanOptics" OceanOptics."OceanOptics" OceanOptics."OceanOptics"] -> w292
          tunnel: [w299 w308 w313 w385 w447 w452 w455 w465] -> w291
          tunnel: w290 -> [_ _ w313 w385 w447 _ w455 w465]
          tunnel: w288 -> [w297 w304 w310 w373 w444 w449 w454 w469]
          tunnel: w287 -> [w298 w305 w312 w374 w445 w450 w462 w470]
          tunnel: [w298 w305 w311 w372 w445 w450 w459 w468] -> w286
          tunnel: [w297 w304 w309 w371 w444 w449 w458 w467] -> w285
          frame "Initialize", Default {
            w296 = 0 ("Motor Position")
            w299 = T8 {"WL Values"=[], "Spectrum Values"=[]}  # clear graph
            n21 = while {
              stop <- w301 stop-if-true
              n22 = global read "GlobalVariables.vi" "Ocean Optics Flag"() -> (w303:bool)
              n23 = global read "GlobalVariables.vi" "Power Meter Flag"() -> (w302:bool)
              n24 = And(x=w303, y=w302) -> (x .and. y?=w301:bool)
            }
            n25 = global write "GlobalVariables.vi" "Motor Position"(w296) -> ()
            n26 = global write "GlobalVariables.vi" "Current Step"(w296) -> ()
          }
          frame "Dark Spec" {
            n27 = global write "GlobalVariables.vi" "Dark Spec Running"(FALSE ("Dark Spec Running")) -> ()
          }
          frame "Wait for Event" {
            n28 = event shown="[2] \"Play Aquisition\": Value Change" {
              selector: _ -> [_ _ _ _ _]
              dyn-events: _ -> [_ _ _ _ _]
              timeout: 10 -> [_ _ _ _ _]
              tunnel: [OceanOptics."OceanOptics" OceanOptics."Clear Dark Spec" OceanOptics."OceanOptics" OceanOptics."Save" OceanOptics."Clear Dark Spec"] -> w315
              tunnel: w312 -> [w318 w321 w327 w335 w338]
              tunnel: w310 -> [w317 w320 w326 w334 w337]
              tunnel: [w318 w321 w325 w335 w338] -> w311
              tunnel: [w317 w320 w324 w334 w337] -> w309
              event Timeout {
                n29 = event-data() -> ()  [unwired: 1 in, 3 out]
              }
              event "Store Dark Spec": Value Change {
                n30 = event-data() -> ()  [unwired: 1 in, 3 out]
                n31 = global write "GlobalVariables.vi" "Dark Spec Running"(TRUE ("Dark Spec Running")) -> ()
              }
              event "Play Aquisition": Value Change {
                w329 = T7 {"Signal State"="", "Step"=0.0, "Integration value"=0.0, "Peak value"=0.0, "Peak Wavelenght"=0.0, "Spectrum values "=[], "Error"={"status"=FALSE, "code"=0, "source"=""}}  # RL-Signal
                # "Mandar Clear Graph"
                n32 = event-data() -> ()  [unwired: 1 in, 3 out]
                n33 = Bundle By Name(cluster=w329, "Signal State"="Clear Graph") -> (w328:T7)
                n34 = Enqueue Element(queue=w327, element=w328, error in (no error)=w326) -> (queue out=w325:refnum<queue>, error out=w324:errorcluster)  [unwired: 1 in, 1 out]
                n35 = global write "GlobalVariables.vi" "Experiment Running"(TRUE ("Experiment Running")) -> ()
                n36 = global write "GlobalVariables.vi" "Step Stop"("Step Stop") -> ()
              }
              event "Save Aquisition": Value Change {
                n37 = event-data() -> ()  [unwired: 1 in, 3 out]
              }
              event "Clear Dark Spec": Value Change {
                n38 = event-data() -> ()  [unwired: 1 in, 3 out]
              }
            }
          }
          frame "OceanOptics" {
            n39 = global read "GlobalVariables.vi" "Motor Position"() -> (→"Current Position":i32)
            n40 = disable-structure shown="Enabled" {
              disable-tunnel: [w416 w418] -> w381
              disable-tunnel: [w414 w419] -> w349
              frame Disabled {
                n41 = call "SpectrumOfLight.vi"("Select Light Source"="Select Light Source") -> ("Spectrum Values"=w416:dbl[], "WL Values"=w414:dbl[])  [unwired: 9 in]
              }
              frame Enabled {
                n42 = while {
                  tunnel: [w423] -> w419
                  tunnel: [w422] -> w418
                  tunnel: [w421] -> w417
                  stop <- w421 stop-if-true
                  n43 = global read "GlobalVariables.vi" "Wavelenght"() -> (w423:dbl[])
                  n44 = global read "GlobalVariables.vi" "Spectrum Values"() -> (w422:dbl[])
                  n45 = global read "GlobalVariables.vi" "Spectrum Ready"() -> (w421:bool)
                }
                n46 = flat-sequence {
                  tunnel: w417 -> [_]
                  frame #0 {
                    n47 = global write "GlobalVariables.vi" "Spectrum Ready"(FALSE ("Spectrum Ready")) -> ()
                  }
                }
              }
            }
            n48 = Unbundle(w385) -> ("Spectrum Values"=w380:dbl[])  [unwired: 1 out]
            n49 = global read "GlobalVariables.vi" "Power Meter"() -> (→"Power Meter [W]" →"Power Meter [W]":dbl)
            n50 = Array Size(array=w380) -> (size(s)=w382:i32)
            n51 = Greater?(x=w382, y=0.0) -> (0:w384:bool)
            n52 = global read "GlobalVariables.vi" "Experiment Running"() -> (→"Running":bool)
            n53 = case shown="True" w384 {
              tunnel: w381 -> [w440 w443]
              tunnel: w380 -> [_ w442]
              tunnel: [w440 w441] -> w340
              frame False {
              }
              frame True {
                n54 = Subtract(x=w443, y=w442) -> (x-y=w441:dbl[])
              }
            }
            n55 = global write "GlobalVariables.vi" "Wavelenght"(w349) -> ()
            n56 = Bundle("Wavelenght"=w349, "Spectrum Values"=w340) -> (w376:T9)  [unwired: 1 in]
            n57 = global read "GlobalVariables.vi" "Dark Spec Running"() -> (w378:bool)
            n58 = case shown="False" w378 {
              tunnel: [OceanOptics."Wait for Event" OceanOptics."Dark Spec"] -> w379
              frame False {
              }
              frame True {
              }
            }
            n59 = for {
              tunnel: w349 -> [w389]
              tunnel: w340 -> [w410]
              tunnel: "Range List" -> [w413] mode=indexing
              tunnel: [w405] -> _ mode=indexing
              tunnel: [w407] -> w351
              tunnel: [w406] -> w354
              tunnel: "threshold" -> [w404]
              tunnel: [w401] -> w350
              tunnel: "width" -> [w394]
              tunnel: [w390] -> w341
              w408 = T10 0 items=["Trapezoidal Rule", "Simpson's Rule", "Simpson's 3/8 Rule", "Bode Rule"] ("integration method")
              n60 = Unbundle By Name(w413) -> ("Name"=w406:string, "Inicial"=w411:dbl, "Final"=w412:dbl)
              n61 = Index Array(array=w389, index #1=1 ("index"), index #2=0 ("index")) -> (element #1=w396:dbl, element #2=w397:dbl)
              n62 = Subtract(x=w396, y=w397) -> (x-y=w395:dbl)
              "delta WL" <- w395
              n63 = call "wavelenghtToindex.vi"("WL in"=w412, "WL Values"=w389) -> ("index of WL"=w409:i32)  [unwired: 9 in]
              n64 = call "wavelenghtToindex.vi"("WL in"=w411, "WL Values"=w389) -> ("index of WL"=w387:i32)  [unwired: 9 in]
              n65 = Subtract(x=w409, y=w387) -> (x-y=w386:i32)
              n66 = Array Subset(array=w410, index=w387, length=w386) -> (w405:dbl[])
              n67 = Array Subset(array=w389, index=w387, length=w386) -> (w388:dbl[])
              n68 = call <vilib>:"Peak Detector.vi"("peaks/valleys"=enum32{"Peaks", "Valleys"}."Peaks", "width"=w394, "threshold"=w404, "X"=w405) -> ("Amplitudes"=w402:dbl[], "Locations"=w393:dbl[])  [unwired: 3 in, 3 out]
              n69 = call-poly <vilib>:"Numeric Integration.vi"("integration method"=w408, "dt"=w395, "Input Array"=w405) -> ("result"=w407:dbl)  [unwired: 1 out]
              n70 = call "locationsToWL.vi"("Locations index"=w393, "WL Values"=w388) -> ("Locations WL"=w391:dbl[])  [unwired: 9 in]
              n71 = Index Array(array=w402, index=0) -> (element=w401:dbl)
              n72 = Index Array(array=w391, index=0) -> (element=w390:dbl)
            }
            n73 = global read "GlobalVariables.vi" "Experiment Running"() -> (w365:bool)
            n74 = global read "GlobalVariables.vi" "Motor moving"() -> (w367:bool)
            n75 = Not(x=w367) -> (.not. x?=w364:bool)
            n76 = And(x=w365, y=w364) -> (x .and. y?=w366:bool)
            n77 = case shown="True" w366 {
              tunnel: w374 -> [w425 w435]
              tunnel: w373 -> [w424 w434]
              tunnel: w340 -> [_ w432]
              tunnel: [w425 w431] -> w372
              tunnel: [w424 w430] -> w371
              tunnel: w351 -> [_ w428]
              tunnel: w341 -> [_ w427]
              tunnel: w350 -> [_ w426]
              frame False {
              }
              frame True {
                w437 = T7 {"Signal State"="", "Step"=0.0, "Integration value"=0.0, "Peak value"=0.0, "Peak Wavelenght"=0.0, "Spectrum values "=[], "Error"={"status"=FALSE, "code"=0, "source"=""}}  # RL-Signal
                n78 = global read "GlobalVariables.vi" "Current Step"() -> (w429:i32)
                n79 = Bundle By Name(cluster=w437, "Integration value"=w428, "Peak Wavelenght"=w427, "Peak value"=w426, "Spectrum values"=w432, "Signal State"="add spectrum", "Step"=w429) -> (w433:T7)
                n80 = Enqueue Element(queue=w435, element=w433, error in (no error)=w434) -> (queue out=w431:refnum<queue>, error out=w430:errorcluster)  [unwired: 1 in, 1 out]
              }
            }
            n81 = Build Array(w341) -> (w353:dbl[])
            n82 = Build Array(w350) -> (w352:dbl[])
            n83 = Bundle(w353, w352) -> (w377:cluster{dbl[], dbl[]})  [unwired: 1 in]
            n84 = Number To Fractional String(number=w351, precision (6)=i16 0) -> (F-format string=w346:string)  [unwired: 2 in]
            n85 = Number To Fractional String(number=w350, precision (6)=i16 0) -> (F-format string=w345:string)  [unwired: 2 in]
            n86 = Number To Fractional String(number=w341, precision (6)=i16 2) -> (F-format string=w342:string)  [unwired: 2 in]
            n87 = Build Array(w376, w377) -> (→"Spectrum":T11)
            n88 = Build Array("Name", "Integration", "Peak", "WL") -> (w360:string[])
            n89 = Build Array(w354, w346, w345, w342) -> (w357:string[])
            n90 = Build Array(w360, w357) -> (→"table":string[][])
          }
          frame "Graph" {
          }
          frame "Clear Dark Spec" {
            w452 = T8 {"WL Values"=[], "Spectrum Values"=[]}  # clear graph
          }
          frame "Create File" {
            w461 = T7 {"Signal State"="", "Step"=0.0, "Integration value"=0.0, "Peak value"=0.0, "Peak Wavelenght"=0.0, "Spectrum values "=[], "Error"={"status"=FALSE, "code"=0, "source"=""}}  # RL-Signal
            n91 = Bundle By Name(cluster=w461, "Signal State"="Create File") -> (w460:T7)
            n92 = Enqueue Element(queue=w462, element=w460, error in (no error)=w454) -> (queue out=w459:refnum<queue>, error out=w458:errorcluster)  [unwired: 1 in, 1 out]
          }
          frame "Save" {
            w472 = T7 {"Signal State"="", "Step"=0.0, "Integration value"=0.0, "Peak value"=0.0, "Peak Wavelenght"=0.0, "Spectrum values "=[], "Error"={"status"=FALSE, "code"=0, "source"=""}}  # RL-Signal
            n93 = Bundle By Name(cluster=w472, "Signal State"="Save") -> (w471:T7)
            n94 = Enqueue Element(queue=w470, element=w471, error in (no error)=w469) -> (queue out=w468:refnum<queue>, error out=w467:errorcluster)  [unwired: 1 in, 1 out]
          }
        }
      }
      n95 = while {
        shift-right: [w159] -> _
        shift-left: PowerMeterSteps."Initialize" ("Enum") -> [w160]
        stop <- FALSE stop-if-true
        # "Power Meter Loop"
        n96 = case shown="\"Get Power\"" w160 {
          tunnel: [PowerMeterSteps."Wait for Event" ("Enum") PowerMeterSteps."Wait for Event" ("Enum") w168 PowerMeterSteps."corrects step" ("Enum") PowerMeterSteps."Wait for Event" ("Enum") PowerMeterSteps."Wait for Event" ("Enum") PowerMeterSteps."Wait for Event" ("Enum")] -> w159
          frame "Initialize", Default {
            n97 = while {
              stop <- w163 stop-if-true
              n98 = global read "GlobalVariables.vi" "Ocean Optics Flag"() -> (w165:bool)
              n99 = global read "GlobalVariables.vi" "Power Meter Flag"() -> (w164:bool)
              n100 = And(x=w165, y=w164) -> (x .and. y?=w163:bool)
            }
          }
          frame "Graph" {
          }
          frame "Wait for Event" {
            n101 = event shown="[5] \"max Power Go\": Value Change" {
              selector: _ -> [_ _ _ _ _ _ _]
              dyn-events: _ -> [_ _ _ _ _ _ _]
              timeout: 10 -> [_ _ _ _ _ _ _]
              tunnel: [PowerMeterSteps."Get Power" ("Enum") w171 w178 PowerMeterSteps."Tuning" ("Enum") PowerMeterSteps."MoveMotor" ("Enum") PowerMeterSteps."MoveMotor" ("Enum") PowerMeterSteps."MoveMotor" ("Enum")] -> w168
              event Timeout {
                n102 = event-data() -> ()  [unwired: 1 in, 3 out]
              }
              event "Power up": Value Change {
                n103 = event-data() -> ()  [unwired: 1 in, 6 out]
                n104 = global read "GlobalVariables.vi" "Motor Steps Max"() -> (w173:i32)
                n105 = global read "GlobalVariables.vi" "Motor Position"() -> (w174:i32)
                n106 = Increment(x=w174) -> (x+1=w170:i32)
                n107 = Greater Or Equal?(x=w170, y=w173) -> (x >= y?=w172:bool)
                n108 = case shown="False" w172 {
                  tunnel: [PowerMeterSteps."MoveMotor" ("Enum") PowerMeterSteps."Wait for Event" ("Enum")] -> w171
                  frame False {
                    n109 = global write "GlobalVariables.vi" "Motor Target"(1.0 ("Motor Target")) -> ()
                  }
                  frame True {
                  }
                }
              }
              event "Power down": Value Change {
                n110 = event-data() -> ()  [unwired: 1 in, 6 out]
                n111 = global read "GlobalVariables.vi" "Motor Position"() -> (w180:i32)
                n112 = Decrement(x=w180) -> (x-1=w182:i32)
                n113 = Less Or Equal?(x=w182, y=0) -> (x <= y?=w181:bool)
                n114 = case shown="False" w181 {
                  tunnel: [PowerMeterSteps."MoveMotor" ("Enum") PowerMeterSteps."Wait for Event" ("Enum")] -> w178
                  frame False {
                    n115 = global write "GlobalVariables.vi" "Motor Target"(-1.0 ("Motor Target")) -> ()
                  }
                  frame True {
                  }
                }
              }
              event "Tuning Motor": Value Change {
                n116 = event-data() -> ()  [unwired: 1 in, 6 out]
              }
              event "min Power": Value Change {
                n117 = event-data() -> ()  [unwired: 1 in, 6 out]
                n118 = global read "GlobalVariables.vi" "Motor Position"() -> (w188:i32)
                n119 = Subtract(x=0, y=w188) -> (x-y=w187:i32)
                n120 = global write "GlobalVariables.vi" "Motor Target"(w187) -> ()
              }
              event "max Power Go": Value Change {
                n121 = event-data() -> ()  [unwired: 1 in, 6 out]
                n122 = global read "GlobalVariables.vi" "Motor Steps Max"() -> (w193:i32)
                n123 = global read "GlobalVariables.vi" "Motor Position"() -> (w192:i32)
                n124 = Subtract(x=w193, y=w192) -> (x-y=w191:i32)
                n125 = global write "GlobalVariables.vi" "Motor Target"(w191) -> ()
              }
              event "Half Power": Value Change {
                n126 = event-data() -> ()  [unwired: 1 in, 6 out]
                n127 = global read "GlobalVariables.vi" "Motor Steps Max"() -> (w199:i32)
                n128 = global read "GlobalVariables.vi" "Motor Position"() -> (w196:i32)
                n129 = Divide(x=w199, y=2) -> (x/y=w197:dbl)
                n130 = Subtract(x=w197, y=w196) -> (x-y=w195:dbl)
                n131 = global write "GlobalVariables.vi" "Motor Target"(w195) -> ()
              }
            }
          }
          frame "Tuning" {
            n132 = while {
              border: dbl[] [] -> [_]
              i -> [w228]
              stop <- w231 stop-if-true
              # "mover motor"
              n133 = flat-sequence {
                tunnel: [w243] -> w221
                tunnel: [w251] -> w222
                tunnel: w221 -> [w251]
                frame #0 {
                  n134 = while {
                    tunnel: [w244] -> w243
                    stop <- w245 stop-if-true
                    n135 = global read "GlobalVariables.vi" "Power Meter"() -> (w244:dbl)
                    n136 = global read "GlobalVariables.vi" "Power Meter Ready"() -> (w245:bool)
                  }
                  "Power Meter" <- w243
                  n137 = local write "Power Meter"(w243) -> ()
                }
                frame #1 {
                  w248 = u16 0 items=["Full step", "Half step", "1/4 step", "1/8 step", "1/16 step", "1/32 step"] ("Step resolution")
                  # "mover motor"
                  n138 = global write "GlobalVariables.vi" "Power Meter Ready"(FALSE ("Power Meter Ready")) -> ()
                  n139 = call "RD_StepMotor_WP.vi"("Step resolution"=w248, "Direction"=TRUE, "Time between steps (ms)"=1, "Steps"=i64 1) -> ()  [unwired: 8 in]
                }
              }
              n140 = disable-structure shown="Disabled" {
                frame Disabled {
                  n141 = call "PoweMeter-Demo.vi"() -> ()  [unwired: 10 in, 2 out]
                }
                frame Enabled {
                }
              }
              n142 = Wait (ms)(milliseconds to wait=u32 5) -> ()  [unwired: 1 out]
              n143 = feedback #1() -> (w242:dbl[])
              n144 = Build Array (concatenate)(w242, w222) -> (w217:dbl[])
              "appended array" <- w217
              n145 = Array Max & Min(array=w217) -> (max value=w219:dbl, min value=w218:dbl)  [unwired: 2 out]
              "Max Power" <- w219
              "Min Power" <- w218
              "Min Power" <- w218
              "Max Power" <- w219
              n146 = Subtract(x=w219, y=w218) -> (x-y=w235:dbl)
              n147 = Divide(x=w235, y=2.0) -> (x/y=w233:dbl)
              n148 = Add(x=w233, y=w218) -> (x+y=w236:dbl)
              n149 = call <vilib>:"Peak Detector.vi"("peaks/valleys"=enum32{"Peaks", "Valleys"}."Valleys", "width"=10 ("width 2"), "threshold"=w236, "X"=w217) -> ("Amplitudes"=→"Amplitudes":dbl[], "Locations"=w216:dbl[], "# found"=w206:i32)  [unwired: 3 in, 2 out]
              "# found" <- w206
              "Locations" <- w216
              n150 = feedback-in #1(w217) -> ()
              n151 = Equal?(x=w206, y=3) -> (x = y?=w231:bool)
              n152 = Decrement(x=w206) -> (x-1=w239:i32)
              n153 = Decrement(x=w206) -> (x-1=w204:i32)
              n154 = for {
                N: w239 -> [_]
                tunnel: w216 -> [w257]
                tunnel: [w253] -> w238 mode=indexing
                tunnel: [w252] -> w227
                i -> [w255]
                n155 = Increment(x=w255) -> (x+1=w256:i32)
                n156 = Index Array(array=w257, index #1=w256, index #2=w255) -> (element #1=w252:dbl, element #2=w254:dbl)
                n157 = Subtract(x=w252, y=w254) -> (x-y=w253:dbl)
              }
              "Array" <- w238
              n158 = Decrement(x=w204) -> (x-1=w205:i32)
              n159 = Index Array(array=w216, index=w205) -> (element=w213:dbl)
              n160 = Index Array(array=w216, index #1=w204, index #2=w205) -> (element #1=w214:dbl, element #2=w215:dbl)
              n161 = Subtract(x=w214, y=w215) -> (x-y=w210:dbl)
              n162 = Add(x=w213, y=0.0) -> (x+y=w212:dbl)
              n163 = Divide(x=w210, y=2.0) -> (x/y=w211:dbl)
              n164 = Array Subset(array=w217, index=w212, length=w211) -> (w203:dbl[])
              "Waveform Graph 2" <- w203
              n165 = Subtract(x=w228, y=w227) -> (x-y=w220:dbl)
              "step error" <- w220
              n166 = call <vilib>:"Std Deviation and Variance.vi"("X"=w238) -> ("mean"=w225:dbl, "standard deviation"=→"standard deviation":dbl)  [unwired: 1 in, 1 out]
              "mean" <- w225
              n167 = Divide(x=w225, y=2.0) -> (x/y=w224:dbl)
              n168 = global write "GlobalVariables.vi" "Power steps curve"(w203) -> ()
              n169 = To Unsigned Long Integer(number=w224) -> (unsigned 32bit integer=w223:u32)
              n170 = Array Size(array=w203) -> (size(s)=→"size(s)":i32)
              n171 = global write "GlobalVariables.vi" "Step error"(w220) -> ()
              n172 = global write "GlobalVariables.vi" "Motor Steps Max"(w223) -> ()
              "Numeric Control" <- w228
            }
          }
          frame "Get Power" {
            n173 = disable-structure shown="Disabled" {
              frame Disabled {
                n174 = call "PoweMeter-Demo.vi"("reset"=TRUE) -> ()  [unwired: 9 in, 2 out]
              }
              frame Enabled {
              }
            }
            n175 = flat-sequence {
              frame #0 {
                n176 = while {
                  stop <- w259 stop-if-true
                  n177 = global read "GlobalVariables.vi" "Power Meter"() -> (→"Power Meter":dbl)
                  n178 = global read "GlobalVariables.vi" "Power Meter Ready"() -> (w259:bool)
                }
              }
              frame #1 {
                n179 = global write "GlobalVariables.vi" "Power Meter Ready"(FALSE ("Power Meter Ready")) -> ()
              }
            }
          }
          frame "MoveMotor" {
            n180 = global read "GlobalVariables.vi" "Motor Position"() -> (w269:i32)
            n181 = global read "GlobalVariables.vi" "Motor Target"() -> (w268:dbl)
            n182 = global read "GlobalVariables.vi" "Motor Steps Max"() -> (w267:i32)
            n183 = Add(x=w269, y=w268) -> (x+y=w265:dbl)
            n184 = Increment(x=w267) -> (x+1=w263:i32)
            n185 = Greater?(x=w268, y=0.0) -> (0:w271:bool)
            n186 = Absolute Value(x=w268) -> (abs(x)=w272:dbl)
            n187 = In Range and Coerce(upper limit=w263, x=w265, lower limit=0) -> (In Range?=w264:bool)  [unwired: 1 out]
            n188 = case shown="True" w264 {
              tunnel: w272 -> [_ w278]
              tunnel: w271 -> [_ w277]
              tunnel: w265 -> [_ w274]
              frame False {
              }
              frame True {
                w276 = u16 0 items=["Full step", "Half step", "1/4 step", "1/8 step", "1/16 step", "1/32 step"] ("Step resolution")
                # "Atualiza posição Motor"
                # "LOOP de Mover o Motor"
                n189 = call "RD_StepMotor_WP.vi"("Step resolution"=w276, "Direction"=w277, "Time between steps (ms)"=10, "Steps"=w278) -> ()  [unwired: 8 in]
                n190 = global write "GlobalVariables.vi" "Motor Position"(w274) -> ()
                n191 = global write "GlobalVariables.vi" "Current Step"(w274) -> ()
                "Motor Target" <- w274
              }
            }
          }
          frame "corrects step" {
            w282 = u16 0 items=["Full step", "Half step", "1/4 step", "1/8 step", "1/16 step", "1/32 step"] ("Step resolution")
            n192 = global read "GlobalVariables.vi" "Step error"() -> (w281:i32)
            n193 = global write "GlobalVariables.vi" "Motor Position"(0 ("Current Step")) -> ()
            n194 = call "RD_StepMotor_WP.vi"("Step resolution"=w282, "Direction"=FALSE, "Time between steps (ms)"=10, "Steps"=w281) -> ()  [unwired: 8 in]
          }
        }
      }
      n195 = while {
        tunnel: w46 -> [w70]
        tunnel: w45 -> [w69]
        shift-right: [w62] -> _
        shift-left: dbl[][] [] -> [w67]
        shift-right: [w57] -> _
        shift-left: w43 -> [w58]
        shift-right: [w55] -> _
        shift-left: w43 -> [w56]
        shift-right: [w53] -> _
        shift-left: w43 -> [w54]
        shift-right: [w51] -> _
        shift-left: dbl[] [] -> [w52]
        stop <- FALSE stop-if-true
        # "Graph Loop"
        n196 = Dequeue Element(queue=w70, error in (no error)=w69) -> (element=w66:T7, error out=w68:errorcluster)  [unwired: 1 in, 2 out]
        n197 = Unbundle By Name(w66) -> ("Integration value"=w61:dbl, "Peak Wavelenght"=w60:dbl, "Peak value"=w59:dbl, "Signal State"=w65:string, "Step"=w63:dbl, "Spectrum values"=w64:dbl[])
        n198 = case shown="\"Save\"" w65 {
          tunnel: w68 -> [_ _ _ _]
          tunnel: w67 -> [w92 _ w121 w158]
          tunnel: w64 -> [w73 _ _ _]
          tunnel: w63 -> [_ _ _ _]
          tunnel: [w91 dbl[][] [] w121 w158] -> w62
          tunnel: w61 -> [w90 _ _ _]
          tunnel: w60 -> [w89 _ _ _]
          tunnel: w59 -> [w88 _ _ _]
          tunnel: w58 -> [w87 _ w118 w157]
          tunnel: [w86 dbl[] [] w118 w157] -> w57
          tunnel: w56 -> [w85 _ w116 w156]
          tunnel: [w84 dbl[] [] w116 w156] -> w55
          tunnel: w54 -> [w83 _ w117 w155]
          tunnel: [w72 dbl[] [] w117 w155] -> w53
          tunnel: w52 -> [w82 _ w119 w154]
          tunnel: [w80 dbl[] [] w119 w154] -> w51
          frame "add spectrum" {
            # "Spectrum values"
            # "Power"
            # "Amplitude"
            # "Location"
            # "Integration"
            n199 = while {
              tunnel: [w98] -> w78
              stop <- w99 stop-if-true
              n200 = global read "GlobalVariables.vi" "Power Meter"() -> (w98:dbl)
              n201 = global read "GlobalVariables.vi" "Power Meter Ready"() -> (w99:bool)
            }
            n202 = flat-sequence {
              tunnel: w78 -> [_]
              tunnel: [w93] -> w77
              frame #0 {
                n203 = global read "GlobalVariables.vi" "Current Step"() -> (w96:i32)
                n204 = global read "GlobalVariables.vi" "Step Stop"() -> (w95:i32)
                n205 = Increment(x=w96) -> (x+1=w93:i32)
                n206 = Greater Or Equal?(x=w93, y=w95) -> (x >= y?=w94:bool)
                n207 = global write "GlobalVariables.vi" "Motor Position"(w93) -> ()
                n208 = global write "GlobalVariables.vi" "Current Step"(w93) -> ()
                n209 = case shown="True" w94 {
                  frame False {
                  }
                  frame True {
                    n210 = global write "GlobalVariables.vi" "Experiment Running"(FALSE ("Experiment Running")) -> ()
                  }
                }
              }
            }
            n211 = Build Array (concatenate)(w92, w73) -> (w91:dbl[][])
            "Spectrum" <- w91
            n212 = Build Array (concatenate)(w87, w90) -> (w86:dbl[])
            "Integration" <- w86
            n213 = Build Array (concatenate)(w85, w89) -> (w84:dbl[])
            "Locations Peaks" <- w84
            n214 = Build Array (concatenate)(w83, w88) -> (w72:dbl[])
            "Amplitudes" <- w72
            n215 = Build Array (concatenate)(w82, w78) -> (w79:dbl[])
            "Power Meter" <- w79
            n216 = flat-sequence {
              tunnel: w77 -> [w101]
              tunnel: w79 -> [w102]
              tunnel: [w102] -> w76
              tunnel: [w101] -> w75
              tunnel: w76 -> [w108]
              tunnel: w75 -> [_]
              tunnel: [w108] -> w74
              tunnel: [w110] -> w80
              tunnel: w74 -> [w110]
              frame #0 {
                n217 = global write "GlobalVariables.vi" "Motor moving"(TRUE ("Motor moving")) -> ()
              }
              frame #1 {
                w105 = u16 0 items=["Full step", "Half step", "1/4 step", "1/8 step", "1/16 step", "1/32 step"] ("Step resolution")
                n218 = global write "GlobalVariables.vi" "Power Meter Ready"(FALSE ("Power Meter Ready")) -> ()
                n219 = call "RD_StepMotor_WP.vi"("Step resolution"=w105, "Direction"=TRUE, "Time between steps (ms)"=1, "Steps"=i64 1) -> ()  [unwired: 8 in]
              }
              frame #2 {
                n220 = global write "GlobalVariables.vi" "Motor moving"(FALSE ("Motor moving")) -> ()
              }
            }
            n221 = Bundle(w79, w72) -> (→"Sample":cluster{dbl[], dbl[]})  [unwired: 1 in]
          }
          frame "Clear Graph" {
          }
          frame "Save" {
            # "Spectrum"
            # "Power"
            # "Amplitude"
            # "Location"
            # "Integration"
            n222 = call <vilib>:"Application Directory.vi"() -> ("Application Directory"=w125:path)
            n223 = Build Path(base path=w125, name or relative path="Data" ("prompt (Create Folder)")) -> (appended path=w124:path)
            n224 = global read "GlobalVariables.vi" "Wavelenght"() -> (w123:dbl[])
            n225 = Build Array(w119, w118, w117, w116) -> (w120:dbl[][])
            n226 = Build Array (concatenate)(w123, w121) -> (w122:dbl[][])
            n227 = stacked-sequence {
              tunnel: w124 -> [w132 w141 _]
              tunnel: w122 -> [w127 _ _]
              tunnel: w120 -> [_ w140 _]
              frame #0 {
                n228 = call "Create Date Time String.vi"() -> ("Date/Time String"=w130:string)  [unwired: 10 in, 1 out]
                n229 = Concatenate Strings("Spectrum Data" ("string"), w130, ".txt" ("string")) -> (w128:string)
                n230 = Build Path(base path=w132, name or relative path=w128) -> (appended path=w136:path)
                n231 = Open/Create/Replace File(file path (use dialog)=w136, operation (0:open)=T6."replace or create", access (0:read/write)=enum16{"read/write", "read-only", "write-only"}."write-only") -> (refnum out=w139:refnum<file>)  [unwired: 3 in, 2 out]
                n232 = Refnum to Path(1:w139) -> (0:w138:path)
                n233 = call-poly <vilib>:"Write To Spreadsheet File.vi"("transpose? (no:F)"=TRUE, "format (%.3f)"="%6f" ("format string"), "2D data"=w127, "file path (dialog if empty)"=w138) -> ()  [unwired: 4 in, 1 out]
              }
              frame #1 {
                n234 = call "Create Date Time String.vi"() -> ("Date/Time String"=w144:string)  [unwired: 10 in, 1 out]
                n235 = Concatenate Strings("Measures Data" ("string"), w144, ".txt" ("string")) -> (w142:string)
                n236 = Build Path(base path=w141, name or relative path=w142) -> (appended path=w149:path)
                n237 = Open/Create/Replace File(file path (use dialog)=w149, operation (0:open)=T6."replace or create", access (0:read/write)=enum16{"read/write", "read-only", "write-only"}."write-only") -> (refnum out=w152:refnum<file>)  [unwired: 3 in, 2 out]
                n238 = Refnum to Path(1:w152) -> (0:w151:path)
                n239 = call-poly <vilib>:"Write To Spreadsheet File.vi"("transpose? (no:F)"=TRUE, "format (%.3f)"="%6f" ("format string"), "2D data"=w140, "file path (dialog if empty)"=w151) -> ()  [unwired: 4 in, 1 out]
              }
              frame #2 {
                n240 = One Button Dialog(message="Saved !!! ") -> ()  [unwired: 1 in, 1 out]
              }
            }
          }
          frame "Reload Settings", Default {
          }
        }
      }
      n241 = Release Queue(queue=w40, error in (no error)=w39) -> (error out=w41:errorcluster)  [unwired: 1 in, 2 out]
      n242 = call <vilib>:"Simple Error Handler.vi"("error in (no error)"=w41) -> ()  [unwired: 4 in, 5 out]
    }
    frame Error {
    }
  }
  n243 = while {
    tunnel: w5 -> [w489]
    tunnel: w4 -> [_]
    tunnel: [w488] -> w11
    stop <- FALSE stop-if-true
    # "Ocean Optics"
    n244 = flat-sequence {
      tunnel: "Average" -> [w492]
      tunnel: "Integration Time" -> [w493]
      tunnel: w489 -> [w494]
      tunnel: "Correct Electrical Dark" -> [w495]
      tunnel: [w495] -> w484
      tunnel: [w494] -> w483
      tunnel: [w493] -> w482
      tunnel: [w492] -> w481
      tunnel: [w491] -> w478
      tunnel: [w501] -> w485
      tunnel: w484 -> [w504]
      tunnel: w483 -> [w502]
      tunnel: w482 -> [w500]
      tunnel: w481 -> [w499]
      tunnel: w478 -> [w496]
      tunnel: [w496] -> w477
      tunnel: [w508] -> w488
      tunnel: w485 -> [w508]
      tunnel: [w506] -> w479
      tunnel: w477 -> [w505]
      tunnel: [w505] -> w476
      frame #0 {
        n245 = Tick Count (ms)() -> (millisecond timer value=w491:u32)
      }
      frame #1 {
        n246 = call "Omni-Driver-Fast-Acquire-AVG.vi"("Average"=w499, "Correct Electrical Dark"=w504, "Spectrometer number"=0, "Integration Time (ms)"=w500, "Wrapper"=w502) -> ("Spectrum Values"=w497:dbl[], "WL Values"=w498:dbl[], "Wrapper Out"=w501:u32)  [unwired: 1 out]
        n247 = global write "GlobalVariables.vi" "Wavelenght"(w498) -> ()
        n248 = global write "GlobalVariables.vi" "Spectrum Values"(w497) -> ()
      }
      frame #2 {
        n249 = global write "GlobalVariables.vi" "Spectrum Ready"(TRUE ("Spectrum Ready")) -> ()
        n250 = Tick Count (ms)() -> (millisecond timer value=w506:u32)
      }
    }
    n251 = Subtract(x=w479, y=w476) -> (x-y=→"Spectrum delay (ms)":u32)
    n252 = Wait (ms)(milliseconds to wait=u32 10) -> ()  [unwired: 1 out]
  }
  n253 = while {
    tunnel: w2 -> [w524]
    tunnel: w1 -> [w519]
    tunnel: [w525] -> w14
    tunnel: [w516] -> w13
    stop <- "Stop" stop-if-true
    # "Get Power"
    # "Power Meter"
    n254 = flat-sequence {
      tunnel: w519 -> [w530]
      tunnel: [w530] -> w518
      tunnel: [w529] -> w514
      frame #0 {
        n255 = Tick Count (ms)() -> (millisecond timer value=w529:u32)
      }
    }
    n256 = Wait (ms)(milliseconds to wait=u32 10) -> ()  [unwired: 1 out]
    n257 = call "TLPM Set Average Time.vi"("error in (no error)"=w518, "Average Time (0.0)"="Average Time (0.0)", "instrument handle"=w524) -> ("error out"=w522:errorcluster, "instrument handle out"=w526:refnum<visa-resource-name>)  [unwired: 7 in]
    n258 = call "TLPM Measure Power.vi"("error in (no error)"=w522, "instrument handle"=w526) -> ("error out"=w520:errorcluster, "Power"=w511:dbl, "instrument handle out"=w525:refnum<visa-resource-name>)  [unwired: 7 in]
    n259 = Divide(x=w511, y="correction factor") -> (x/y=w509:dbl)
    "Power Value" <- w509
    n260 = flat-sequence {
      tunnel: w520 -> [w532]
      tunnel: [w532] -> w517
      frame #0 {
        n261 = global write "GlobalVariables.vi" "Power Meter Ready"(TRUE ("Power Meter Ready")) -> ()
      }
    }
    n262 = global write "GlobalVariables.vi" "Power Meter"(w509) -> ()
    n263 = flat-sequence {
      tunnel: w517 -> [w528]
      tunnel: [w528] -> w516
      tunnel: [w527] -> w515
      frame #0 {
        n264 = Tick Count (ms)() -> (millisecond timer value=w527:u32)
      }
    }
    n265 = Subtract(x=w515, y=w514) -> (x-y=→"P Meter Delay (ms)":u32)
  }
  n266 = call "Omni-Driver-Fast-Close.vi"("Wrapper In"=w11) -> ()  [unwired: 1 in]
  n267 = call "TLPM Close.vi"("error in (no error)"=w13, "instrument handle"=w14) -> ("error out"=w12:errorcluster)  [unwired: 9 in]
  n268 = flat-sequence {
    tunnel: w12 -> [_]
    frame #0 {
      n269 = Stop() -> ()  [unwired: 1 in]
    }
  }
